vi "toFahrenheit.vi"(11 "y":dbl) -> (3 "Numeric":dbl)   [LabVIEW 2014]
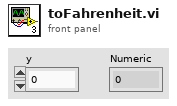
[diagram p1: front panel]
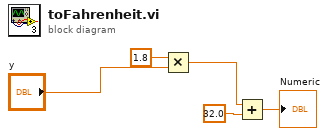
[diagram p0: block diagram]
diagram:
  n1 = Multiply(x=1.8, y="y") -> (x*y=w2:dbl)
  n2 = Add(x=w2, y=32.0) -> (x+y=→"Numeric":dbl)
